vi "UpdateScanControl.vi"(8 "error in (no error)":errorcluster, 11 "Experiment in":refnum<class "Experiment.lvclass">) -> (0 "error out":errorcluster, 3 "Experiment out":refnum<class "Experiment.lvclass">)   [LabVIEW 2014, in "Experiment.lvclass"]
uses:
  Experiment.lvclass
  Experiment.lvclass/Experiment.ctl
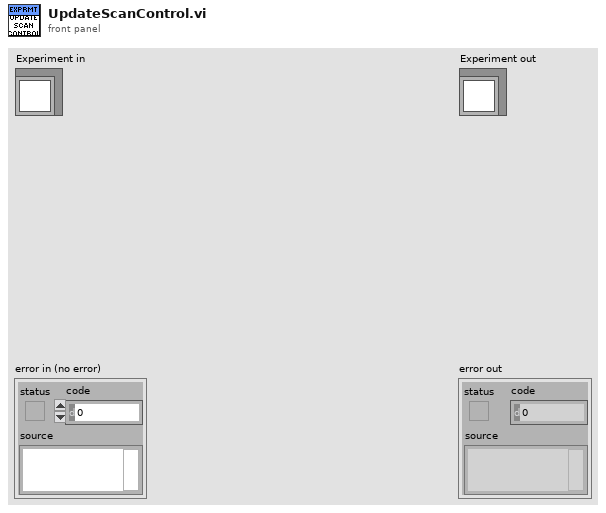
[diagram p1: front panel]
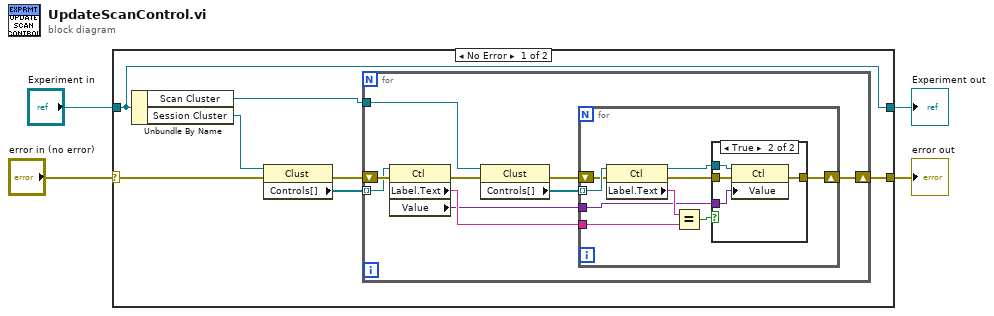
[diagram p0: block diagram]
diagram:
  n1 = case shown="No Error" "error in (no error)" {
    selector: "error in (no error)" -> [w8 w36]
    tunnel: [w7 w36] -> w3
    tunnel: [w6 w35] -> w1
    tunnel: "Experiment in" -> [w6 w35]
    frame No Error {
      n2 = Unbundle By Name(w6) -> ("Scan Cluster"=w9:refnum<vi>, "Session Cluster"=w11:refnum<vi>)
      n3 = property class="Clust"(reference=w11, error in=w8) -> (error out=w10:errorcluster, "Controls[]"=w5:refnum<vi>[])  [unwired: 1 out]
      n4 = for {
        shift-right: [w16] -> w7
        shift-left: w10 -> [w20]
        tunnel: w9 -> [w15]
        tunnel: w5 -> [w12] mode=indexing
        n5 = property class="Ctl"(reference=w12, error in=w20) -> (error out=w14:errorcluster, "Label.Text"=w18:string, "Value"=w17:variant)  [unwired: 1 out]
        n6 = property class="Clust"(reference=w15, error in=w14) -> (error out=w13:errorcluster, "Controls[]"=w19:refnum<vi>[])  [unwired: 1 out]
        n7 = for {
          tunnel: w19 -> [w29] mode=indexing
          shift-right: [w23] -> w16
          shift-left: w13 -> [w25]
          tunnel: w18 -> [w22]
          tunnel: w17 -> [w21]
          n8 = property class="Ctl"(reference=w29, error in=w25) -> (reference out=w28:refnum<vi>, error out=w24:errorcluster, "Label.Text"=w26:string)
          n9 = Equal?(x=w26, y=w22) -> (x = y?=w27:bool)
          n10 = case shown="True" w27 {
            tunnel: w28 -> [_ w34]
            tunnel: w24 -> [w30 w33]
            tunnel: [w30 w32] -> w23
            tunnel: w21 -> [_ w31]
            frame False {
            }
            frame True {
              n11 = property class="Ctl"(reference=w34, error in=w33, "Value"=w31) -> (error out=w32:errorcluster)  [unwired: 1 out]
            }
          }
        }
      }
    }
    frame Error {
    }
  }
  "error out" <- w3
  "Experiment out" <- w1
